vi "XASPage.vi"(7 "LabVIEW Web Service Request":refnum<class "Web Request.lvclass">) -> ()   [LabVIEW 2018]
uses:
  <vilib>/wsapi/Web Request.lvclass
  Type def XSApage.ctl
panel:
  # "Use the Web Service Request input terminal to call the VIs on the Web Services palette. Do not remove it from the connector pane unless you don't need access to the palette."
  # "Each additional control wired to the connector pane will be available as an input in the URL. To include an indicator in terminal-mode output (the default setting), it must also be wired to the connector pane."
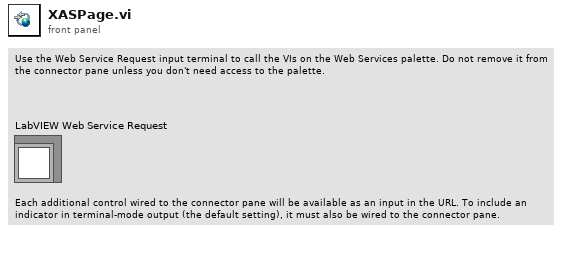
[diagram p1: front panel]
types:
  T1 = typedef "Type def XSApage.ctl" = cluster{"XAS Status":bool, "XAS Mode":u8, "Current Amp Status":bool, "FL Dead Time":dbl, "NAS Connection":bool, "Energy Mode":u8, "Macro Mode":bool, "E0":dbl, "Emin":dbl, "Emax":dbl, "File Name":string, "Queue Name":string, "Current Queue":u8, "Current Scan":u8, "Number of Queue":u8, "Number of scan":u8, "Percent Complete":dbl, "Error Message":string, "Currente Energy":dbl, "I0":u32, "I1":u32, "I2":u32, "If":u32, "In(I0/I1)":dbl, "In(I1/I2)":dbl, "If/I0":dbl, "Start":string, "Finish":string}
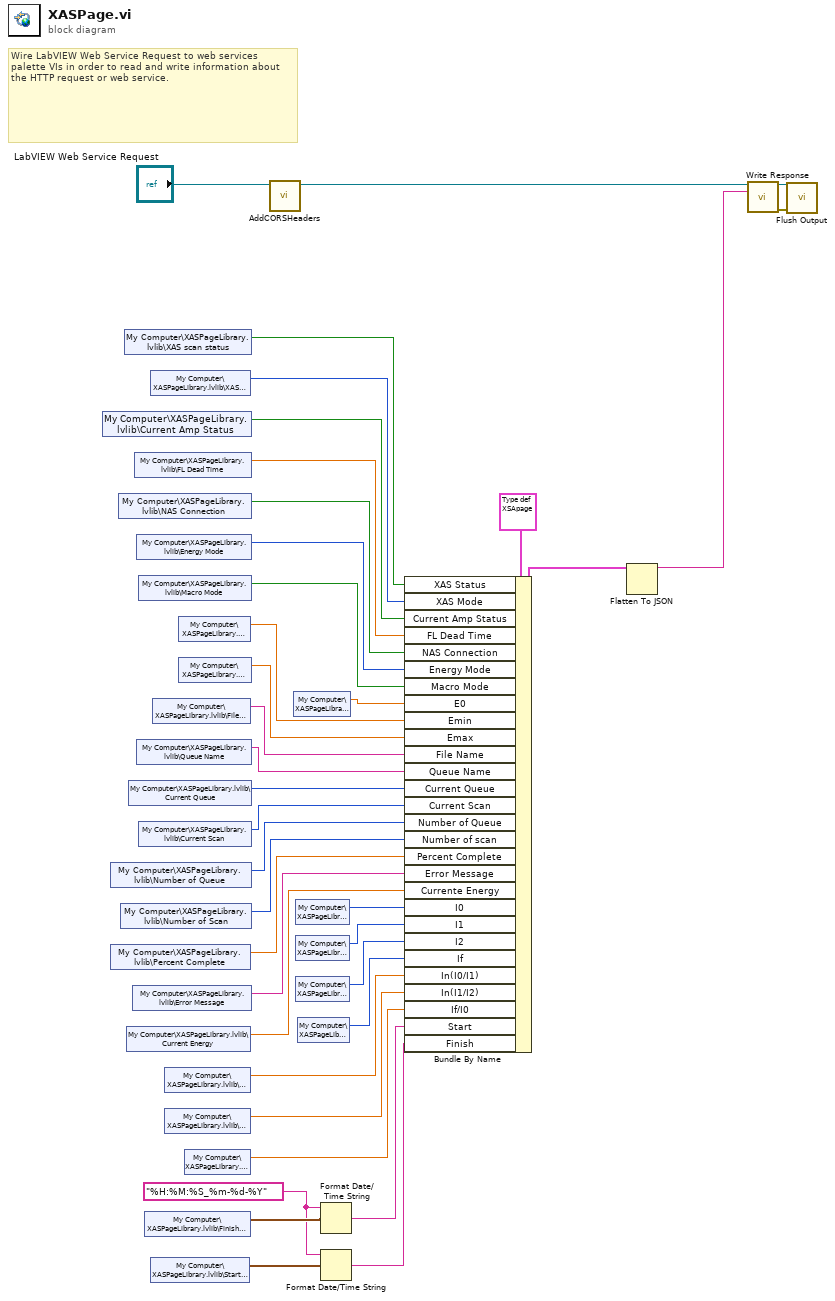
[diagram p0: block diagram]
diagram:
  w1 = "%H:%M:%S_%m-%d-%Y" ("time format string (%c)")
  # "Wire LabVIEW Web Service Request to web services palette VIs in order to read and write information about the HTTP request or web service."
  n1 = shared-variable "My Computer\\XASPageLibrary.lvlib\\Current Amp Status"() -> (w30:bool)  [unwired: 1 in, 1 out]
  n2 = shared-variable "My Computer\\XASPageLibrary.lvlib\\Number of Queue"() -> (w17:u8)  [unwired: 1 in, 1 out]
  n3 = shared-variable "My Computer\\XASPageLibrary.lvlib\\Percent Complete"() -> (w15:dbl)  [unwired: 1 in, 1 out]
  n4 = shared-variable "My Computer\\XASPageLibrary.lvlib\\NAS Connection"() -> (w27:bool)  [unwired: 1 in, 1 out]
  n5 = shared-variable "My Computer\\XASPageLibrary.lvlib\\Number of Scan"() -> (w16:u8)  [unwired: 1 in, 1 out]
  n6 = shared-variable "My Computer\\XASPageLibrary.lvlib\\XAS scan status"() -> (w33:bool)  [unwired: 1 in, 1 out]
  n7 = shared-variable "My Computer\\XASPageLibrary.lvlib\\Current Energy"() -> (w13:dbl)  [unwired: 1 in, 1 out]
  n8 = shared-variable "My Computer\\XASPageLibrary.lvlib\\Current Queue"() -> (w19:u8)  [unwired: 1 in, 1 out]
  n9 = shared-variable "My Computer\\XASPageLibrary.lvlib\\Error Message"() -> (w14:string)  [unwired: 1 in, 1 out]
  n10 = shared-variable "My Computer\\XASPageLibrary.lvlib\\FL Dead Time"() -> (w28:dbl)  [unwired: 1 in, 1 out]
  n11 = shared-variable "My Computer\\XASPageLibrary.lvlib\\Energy Mode"() -> (w26:u8)  [unwired: 1 in, 1 out]
  n12 = shared-variable "My Computer\\XASPageLibrary.lvlib\\Queue Name"() -> (w20:string)  [unwired: 1 in, 1 out]
  n13 = shared-variable "My Computer\\XASPageLibrary.lvlib\\Macro Mode"() -> (w25:bool)  [unwired: 1 in, 1 out]
  n14 = shared-variable "My Computer\\XASPageLibrary.lvlib\\Current Scan"() -> (w18:u8)  [unwired: 1 in, 1 out]
  n15 = shared-variable "My Computer\\XASPageLibrary.lvlib\\Finish Time"() -> (w5:timestamp)  [unwired: 1 in, 1 out]
  n16 = shared-variable "My Computer\\XASPageLibrary.lvlib\\XAS Mode"() -> (w29:u8)  [unwired: 1 in, 1 out]
  n17 = shared-variable "My Computer\\XASPageLibrary.lvlib\\Start Time"() -> (w4:timestamp)  [unwired: 1 in, 1 out]
  n18 = shared-variable "My Computer\\XASPageLibrary.lvlib\\File Name"() -> (w21:string)  [unwired: 1 in, 1 out]
  n19 = shared-variable "My Computer\\XASPageLibrary.lvlib\\In(I0-I1)"() -> (w8:dbl)  [unwired: 1 in, 1 out]
  n20 = shared-variable "My Computer\\XASPageLibrary.lvlib\\In(I1-I2)"() -> (w7:dbl)  [unwired: 1 in, 1 out]
  n21 = shared-variable "My Computer\\XASPageLibrary.lvlib\\Emin"() -> (w23:dbl)  [unwired: 1 in, 1 out]
  n22 = shared-variable "My Computer\\XASPageLibrary.lvlib\\Emax"() -> (w22:dbl)  [unwired: 1 in, 1 out]
  n23 = shared-variable "My Computer\\XASPageLibrary.lvlib\\If-I0"() -> (w6:dbl)  [unwired: 1 in, 1 out]
  n24 = call "AddCORSHeaders.vi"("Web Request in"="LabVIEW Web Service Request") -> ("Web Request out"=w32:refnum<class "Web Request.lvclass">)  [unwired: 10 in]
  n25 = shared-variable "My Computer\\XASPageLibrary.lvlib\\E0"() -> (w24:dbl)  [unwired: 1 in, 1 out]
  n26 = shared-variable "My Computer\\XASPageLibrary.lvlib\\I0"() -> (w12:u32)  [unwired: 1 in, 1 out]
  n27 = shared-variable "My Computer\\XASPageLibrary.lvlib\\I1"() -> (w11:u32)  [unwired: 1 in, 1 out]
  n28 = shared-variable "My Computer\\XASPageLibrary.lvlib\\I2"() -> (w10:u32)  [unwired: 1 in, 1 out]
  n29 = shared-variable "My Computer\\XASPageLibrary.lvlib\\If"() -> (w9:u32)  [unwired: 1 in, 1 out]
  n30 = Format Date/Time String(time format string (%c)=w1, seconds (now)=w5) -> (date/time string=w3:string)  [unwired: 1 in]
  n31 = Format Date/Time String(time format string (%c)=w1, seconds (now)=w4) -> (date/time string=w2:string)  [unwired: 1 in]
  n32 = Bundle By Name(cluster=T1 {"XAS Status"=FALSE, "XAS Mode"=0, "Current Amp Status"=FALSE, "FL Dead Time"=0.0, "NAS Connection"=FALSE, "Energy Mode"=0, "Macro Mode"=FALSE, "E0"=0.0, "Emin"=0.0, "Emax"=0.0, "File Name"="", "Queue Name"="", "Current Queue"=0, "Current Scan"=0, "Number of Queue"=0, "Number of scan"=0, "Percent Complete"=0.0, "Error Message"="", "Currente Energy"=0.0, "I0"=0, "I1"=0, "I2"=0, "If"=0, "In(I0/I1)"=0.0, "In(I1/I2)"=0.0, "If/I0"=0.0, "Start"="", "Finish"=""}, "XAS Status"=w33, "XAS Mode"=w29, "Current Amp Status"=w30, "FL Dead Time"=w28, "NAS Connection"=w27, "Energy Mode"=w26, "Macro Mode"=w25, "E0"=w24, "Emin"=w23, "Emax"=w22, "File Name"=w21, "Queue Name"=w20, "Current Queue"=w19, "Current Scan"=w18, "Number of Queue"=w17, "Number of scan"=w16, "Percent Complete"=w15, "Error Message"=w14, "Currente Energy"=w13, "I0"=w12, "I1"=w11, "I2"=w10, "If"=w9, "In(I0/I1)"=w8, "In(I1/I2)"=w7, "If/I0"=w6, "Start"=w3, "Finish"=w2) -> (w35:T1)
  n33 = Flatten To JSON(anything=w35) -> (JSON string=w34:string)  [unwired: 2 in, 1 out]
  n34 = call <vilib>:"Write Response.vi"("LabVIEW Web Service Request"=w32, "response string"=w34) -> ("LabVIEW Web Service Request out"=w37:refnum<class "Web Request.lvclass">, "error out"=w36:errorcluster)  [unwired: 12 in]
  n35 = call <vilib>:"Flush Output.vi"("LabVIEW Web Service Request"=w37, "error in (no error)"=w36) -> ()  [unwired: 12 in, 2 out]
